vi "Create Object.vi"(10 "Nest Actor":refnum<class "LVCAM.lvclass">) -> (3 "LVCAM Nest Destroyed Msg out":refnum<class "LVCAM Nest Destroyed Msg.lvclass">)   [LabVIEW 2021, in "LVCAM Nest Destroyed.lvlib" / "LVCAM Nest Destroyed Msg.lvclass"]
uses:
  LVCAM Nest Destroyed Msg.lvclass
  LVCAM/LVCAM/LVCAM.lvclass
  LVCAM Nest Destroyed Msg.lvclass/LVCAM Nest Destroyed Msg.ctl
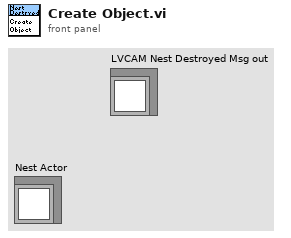
[diagram p1: front panel]
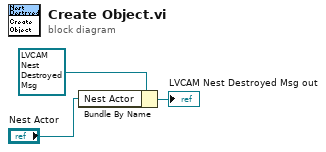
[diagram p0: block diagram]
diagram:
  n1 = Bundle By Name(cluster=refnum<class "LVCAM Nest Destroyed Msg.lvclass"> refnum ("Last Ack Msg in"), "Nest Actor"="Nest Actor") -> (→"LVCAM Nest Destroyed Msg out":refnum<class "LVCAM Nest Destroyed Msg.lvclass">)
